vi "Generate Test Pattern.vi"(8 "error in":errorcluster, 10 "Output Channel":tag="6366/ao0") -> (0 "error out":errorcluster)   [LabVIEW 2024]
uses:
  <vilib>/measure/NI_MABase.lvlib
  <resource>/objmgr/daqmx.rc
  <vilib>/DAQmx/create/channels.llb/DAQmx Create Channel (AO-Voltage-Basic).vi
  <vilib>/DAQmx/write.llb/DAQmx Write (Analog 1D Wfm NChan NSamp).vi
  <vilib>/DAQmx/configure/timing.llb/DAQmx Timing (Sample Clock).vi
panel:
  in  "Offset":dbl=2.5 format="%0.2p"
  in  "amplitude 2":dbl format="%0.2p"
  in  "Clock source":tag="OnboardClock"
  out "Done":bool
  out "SampClk.Rate":dbl format="%#_6p"
  in  "Number of samples":dbl=2000.0 format="%#_8p"
  in  "Sampling rate":dbl=2000000.0 format="%.2p"
  in  "amplitude":dbl=2.5 format="%0.2p"
  in  "frequency":dbl=1000.0 format="%#_6pHz"
  in  "signal type":T1(ring)=enum."Square Wave"
  in  "Range":dbl=10.0 format="%#_6pV"
  out "Waveform Graph":waveform(dbl)[](graph)
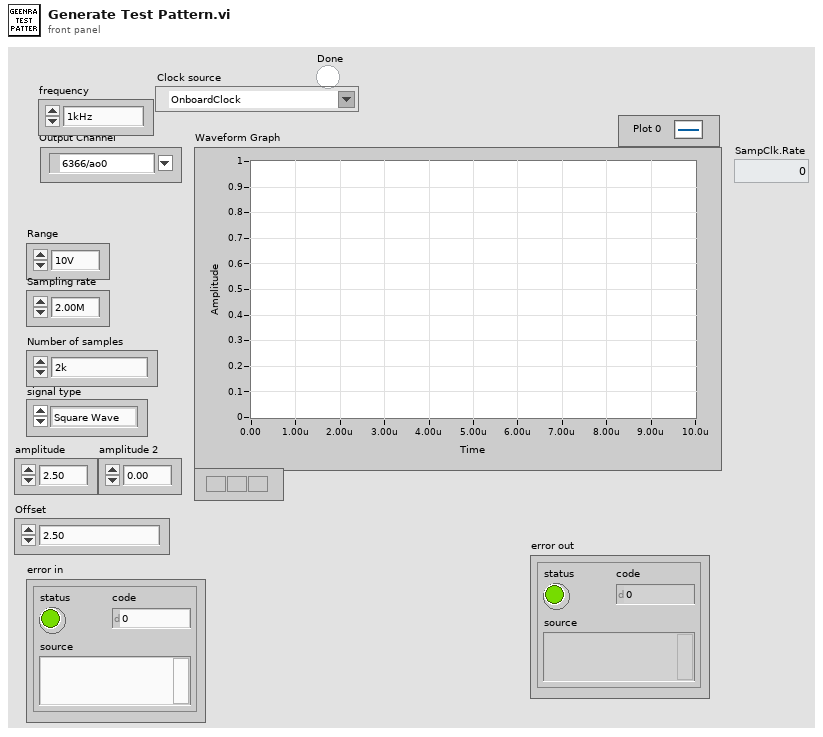
[diagram p1: front panel]
types:
  T1 = enum16{"Sine Wave", "Triangle Wave", "Square Wave", "Sawtooth Wave"}
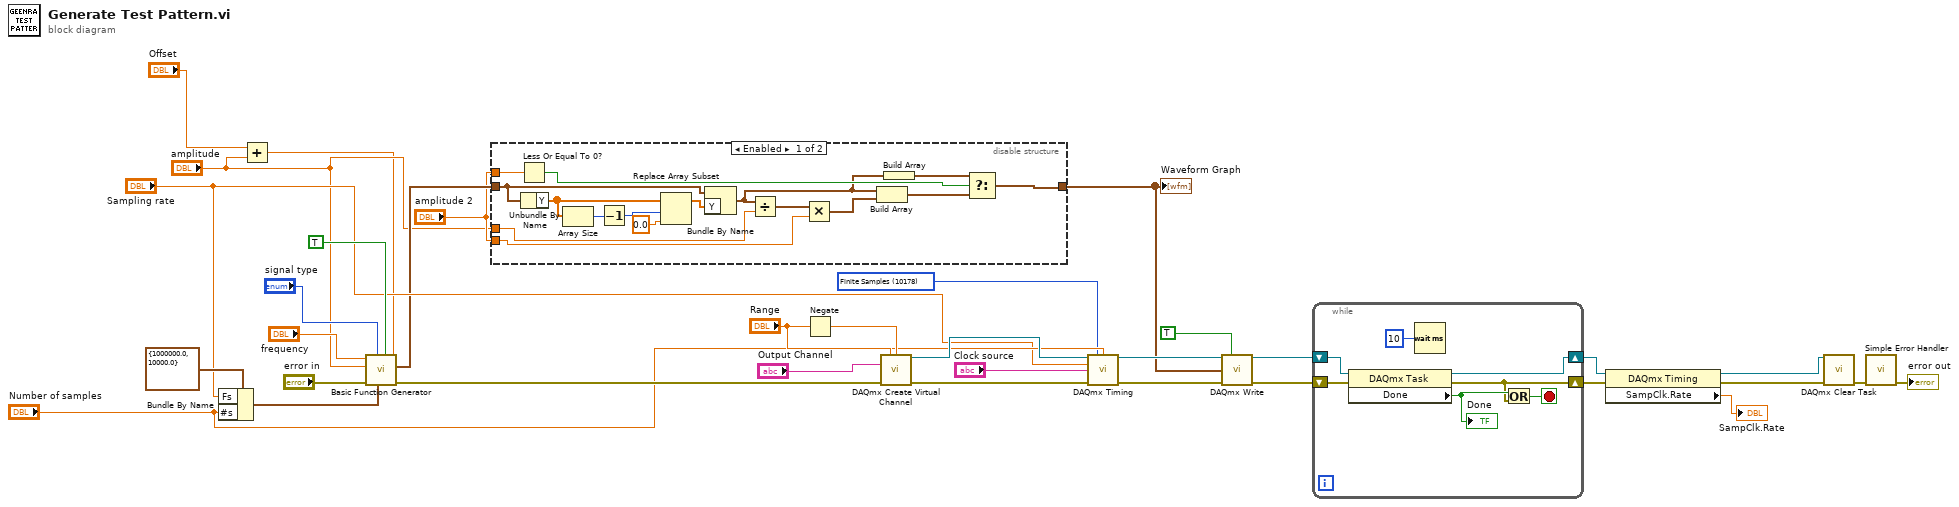
[diagram p0: block diagram]
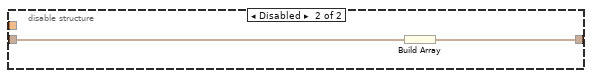
[diagram p2: hidden frame]
diagram:
  w13 = 10178 items=["Finite Samples"=10178, "Continuous Samples"=10123, "Hardware Timed Single Point"=12522] ("sample mode")
  n1 = Bundle By Name(cluster=cluster{"Fs":dbl, "#s":dbl} {"Fs"=1000000.0, "#s"=10000.0} ("sampling info"), "Fs"="Sampling rate", "#s"="Number of samples") -> (w26:cluster{"Fs":dbl, "#s":dbl})
  n2 = Add(x="Offset", y="amplitude") -> (x+y=w1:dbl)
  n3 = call <vilib>:"Basic Function Generator.vi"("offset"=w1, "reset signal"=TRUE, "sampling info"=w26, "signal type"="signal type", "error in (no error)"="error in", "amplitude"="amplitude", "frequency"="frequency") -> ("error out"=w28:errorcluster, "signal out"=w7:waveform(dbl))  [unwired: 2 in, 1 out]
  n4 = disable-structure shown="Enabled" {
    disable-tunnel: w7 -> [w50 w52]
    disable-tunnel: [w35 w51] -> w6
    disable-tunnel: "amplitude" -> [w43 _]
    disable-tunnel: "amplitude 2" -> [w41 _]
    disable-tunnel: "amplitude 2" -> [w40 _]
    frame Enabled {
      n5 = Less Or Equal To 0?(x=w40) -> (x <= 0?=w39:bool)
      n6 = Unbundle By Name(w50) -> ("Y"=w48:dbl[])
      n7 = Array Size(array=w48) -> (size(s)=w49:i32)
      n8 = Decrement(x=w49) -> (x-1=w47:i32)
      n9 = Replace Array Subset(array=w48, new element=0.0 ("new element/subarray"), index=w47) -> (w45:dbl[])
      n10 = Bundle By Name(cluster=w50, "Y"=w45) -> (w38:waveform(dbl))
      n11 = Divide(x=w38, y=w43) -> (x/y=w42:waveform(dbl))
      n12 = Multiply(x=w42, y=w41) -> (x*y=w37:waveform(dbl))
      n13 = Build Array(w38, w37) -> (w36:waveform(dbl)[])
      n14 = Build Array(w38) -> (w44:waveform(dbl)[])
      n15 = Select(t=w44, s=w39, f=w36) -> (s? t:f=w35:waveform(dbl)[])
    }
    frame Disabled {
      n16 = Build Array(w52) -> (w51:waveform(dbl)[])
    }
  }
  "Waveform Graph" <- w6
  n17 = Negate(x="Range") -> (-x=w33:dbl)
  n18 = call-poly <vilib>:"DAQmx Create Virtual Channel.vi"("maximum value"="Range", "minimum value"=w33, "physical channels"="Output Channel", "error in"=w28) -> ("task out"=w20:refnum<k21>, "error out"=w17:errorcluster)  [unwired: 10 in]
  n19 = call-poly <vilib>:"DAQmx Timing.vi"("task/channels in"=w20, "sample mode"=w13, "samples per channel"="Number of samples", "rate"="Sampling rate", "source"="Clock source", "error in"=w17) -> ("task out"=w19:refnum<k21>, "error out"=w16:errorcluster)  [unwired: 8 in]
  n20 = call-poly <vilib>:"DAQmx Write.vi"("task/channels in"=w19, "auto start"=TRUE, "data"=w6, "error in"=w16) -> ("task out"=w12:refnum<k21>, "error out"=w11:errorcluster)  [unwired: 9 in, 1 out]
  n21 = while {
    shift-right: [w58] -> w8
    shift-left: w12 -> [w59]
    shift-right: [w53] -> w9
    shift-left: w11 -> [w57]
    stop <- w54 stop-if-true
    n22 = property class="DAQmx Task"(reference=w59, error in=w57) -> (reference out=w58:refnum<k21>, error out=w53:errorcluster, "Done"=w55:bool)
    "Done" <- w55
    n23 = Wait (ms)(milliseconds to wait=u32 10) -> ()  [unwired: 1 out]
    n24 = Or(x=w55, y=w53) -> (x .or. y?=w54:bool)
  }
  n25 = property class="DAQmx Timing"(reference=w8, error in=w9) -> (reference out=w22:refnum<k21>, error out=w23:errorcluster, "SampClk.Rate"=→"SampClk.Rate":dbl)
  n26 = call <vilib>:"DAQmx Clear Task.vi"("task in"=w22, "error in"=w23) -> ("error out"=w25:errorcluster)  [unwired: 13 in]
  n27 = call <vilib>:"Simple Error Handler.vi"("error in (no error)"=w25) -> ("error out"=→"error out":errorcluster)  [unwired: 4 in, 4 out]
